vi "GetXL_WorkSheetName.vi"(8 "error in (no error)":errorcluster, 11 "Refnum Cluster in":T1) -> (0 "error out":errorcluster, 2 "Name":string, 3 "Refnum Cluster Out":T1)   [LabVIEW 2017, in "excel_configuration.lvlib"]
uses:
  excel_configuration.lvlib
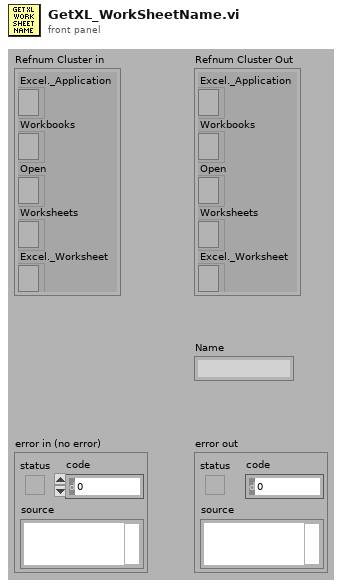
[diagram p1: front panel]
types:
  T1 = cluster{"Excel._Application":refnum<k7>, "Workbooks":refnum<k7>, "Open":refnum<k7>, "Worksheets":refnum<k7>, "Excel._Worksheet":refnum<k7>}
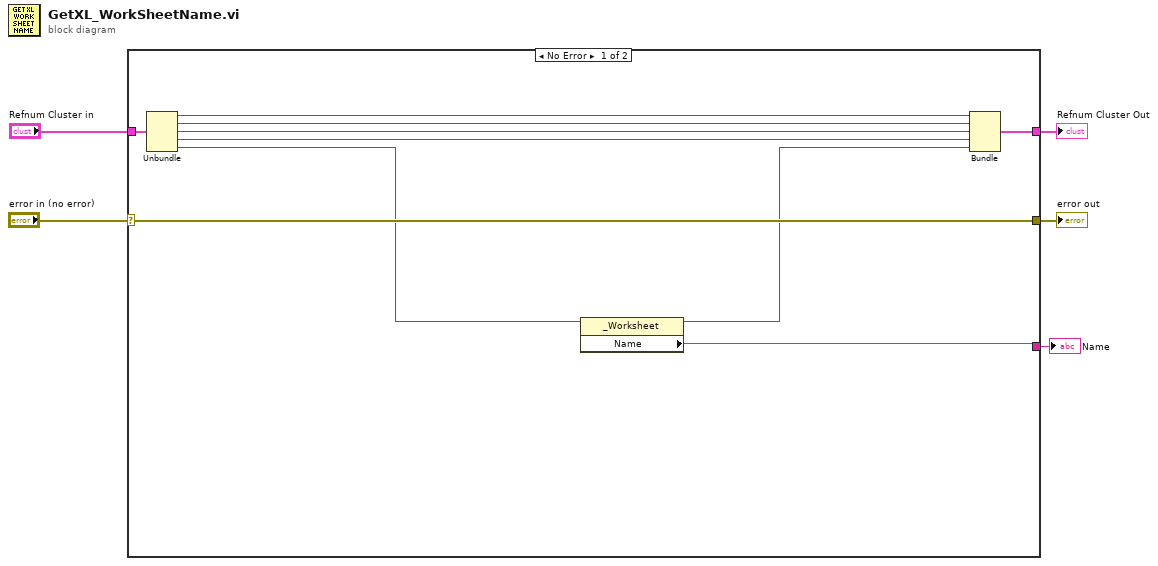
[diagram p0: block diagram]
diagram:
  n1 = case shown="No Error" "error in (no error)" {
    selector: "error in (no error)" -> [w9 w17]
    tunnel: [w12 w16] -> w5
    tunnel: "Refnum Cluster in" -> [w11 w16]
    tunnel: [w9 w17] -> w2
    tunnel: [w6 _] -> w1
    frame No Error {
      n2 = Unbundle(w11) -> ("Excel._Application"=w13:refnum<k7>, "Workbooks"=w14:refnum<k7>, "Open"=w15:refnum<k7>, "Worksheets"=w10:refnum<k7>, "Excel._Worksheet"=w8:refnum<k7>)
      n3 = property class="_Worksheet"(reference=w8) -> (reference out=w7:refnum<k7>, "Name"=w6:string)  [unwired: 1 in, 1 out]
      n4 = Bundle("Excel._Application"=w13, "Workbooks"=w14, "Open"=w15, "Worksheets"=w10, "Excel._Worksheet"=w7) -> (w12:T1)  [unwired: 1 in]
    }
    frame Error {
    }
  }
  "error out" <- w2
  "Refnum Cluster Out" <- w5
  "Name" <- w1
